vi "Unwrap Message.vi"(8 "error in (no error)":errorcluster, 11 "Message in":refnum<class "Message.lvclass">) -> (0 "error out":errorcluster, 1 "Data":variant, 2 "Message":string, 3 "Message out":refnum<class "Message.lvclass">, 4 "Sender":string, 5 "Time Sent":timestamp)   [LabVIEW 2018, in "Application.lvlib" / "Message.lvclass"]
uses:
  Message.lvclass
  Message.lvclass/Message.ctl
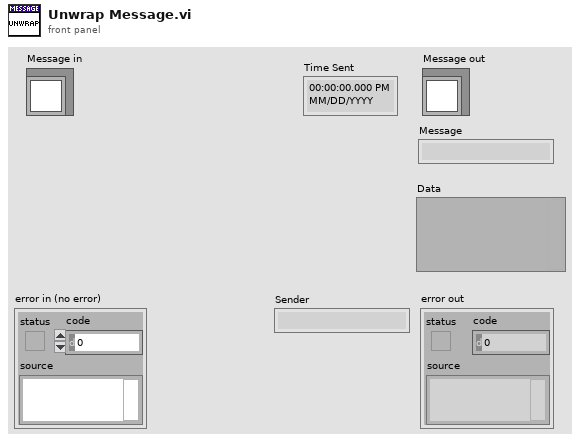
[diagram p1: front panel]
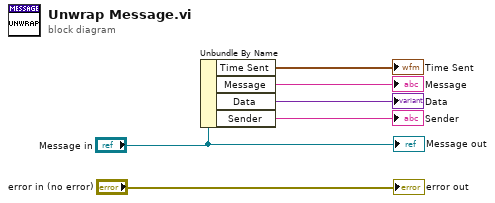
[diagram p0: block diagram]
diagram:
  n1 = Unbundle By Name("Message in") -> ("Time Sent"=→"Time Sent":timestamp, "Message"=→"Message":string, "Data"=→"Data":variant, "Sender"=→"Sender":string)
  "error out" <- "error in (no error)"
  "Message out" <- "Message in"
